vi "1.1odb.vi"() -> ()   [LabVIEW 2020]
panel:
  out "Waveform Chart":i32(graph)
  out "String":string
  out "Numeric":i32
  in  "stop":bool
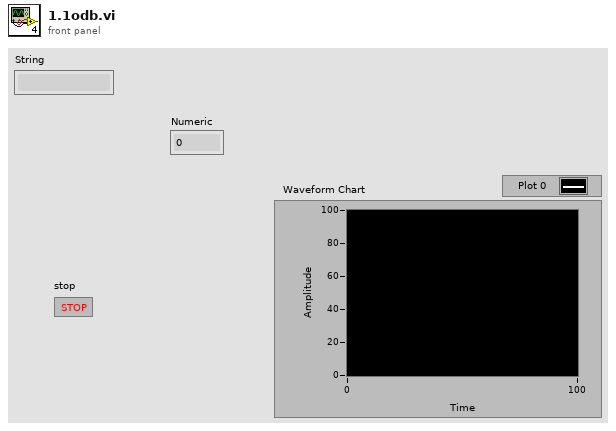
[diagram p1: front panel]
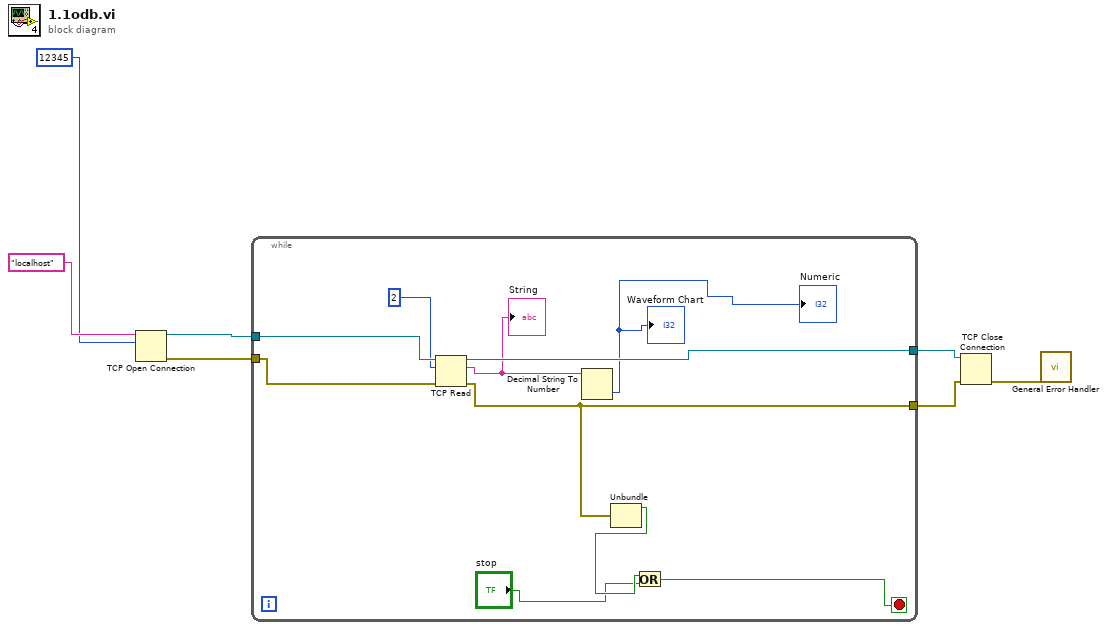
[diagram p0: block diagram]
diagram:
  n1 = TCP Open Connection(address="localhost", remote port or service name=12345) -> (connection ID=w6:refnum<k5>, error out=w7:errorcluster)  [unwired: 3 in]
  n2 = while {
    tunnel: w6 -> [w17]
    tunnel: w7 -> [w15]
    tunnel: [w14] -> w4
    tunnel: [w13] -> w3
    stop <- w10 stop-if-true
    n3 = TCP Read(connection ID=w17, bytes to read=2, error in (no error)=w15) -> (connection ID out=w14:refnum<k5>, data out=w9:string, error out=w13:errorcluster)  [unwired: 2 in]
    "String" <- w9
    n4 = Decimal String To Number(string=w9) -> (number=→"Numeric" →"Waveform Chart":i32)  [unwired: 2 in, 1 out]
    n5 = Unbundle(w13) -> ("status"=w12:bool)  [unwired: 2 out]
    n6 = Or(x=w12, y="stop") -> (x .or. y?=w10:bool)
  }
  n7 = TCP Close Connection(connection ID=w4, error in (no error)=w3) -> (error out=w2:errorcluster)  [unwired: 1 in, 1 out]
  n8 = call <vilib>:"General Error Handler.vi"("error in (no error)"=w2) -> ()  [unwired: 10 in, 5 out]
